vi "mcl_panel_register_events.vi"(8 "error in (no error)":errorcluster, 11 "thorlabs_panel in":refnum<class "mcl_panel.lvclass">) -> (0 "error out":errorcluster, 2 "event_refs cluster":T1, 3 "thorlabs_panel out":refnum<class "mcl_panel.lvclass">)   [LabVIEW 2015, in "mcl_panel.lvclass"]
uses:
  mcl_panel.lvclass
  Thorlabs Kinesis/thorlabs_panel/thorlabs_event_refs.ctl
  Thorlabs Kinesis/thorlabs_panel/thorlabs_events.ctl
  mcl_panel.lvclass/mcl_panel.ctl
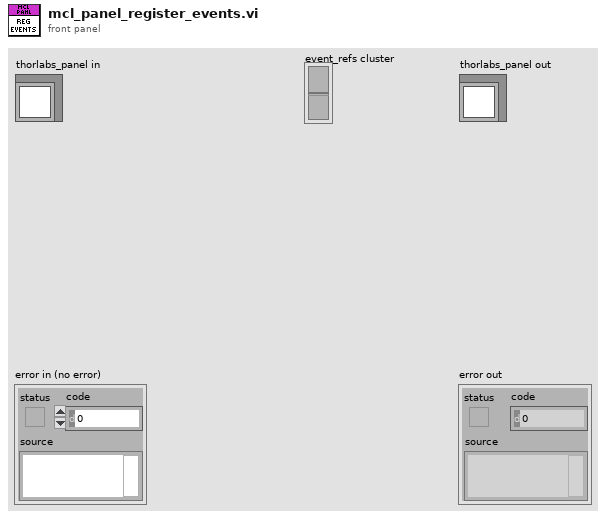
[diagram p1: front panel]
types:
  T1 = typedef "thorlabs_event_refs.ctl" = cluster{"Event Registration Refnum":refnum<event-registration>, "Event Registration Refnum":refnum<event-registration>}
  T2 = typedef "thorlabs_events.ctl" = cluster{"mcl_status":refnum<user-event>, "piezo_positions":refnum<user-event>}
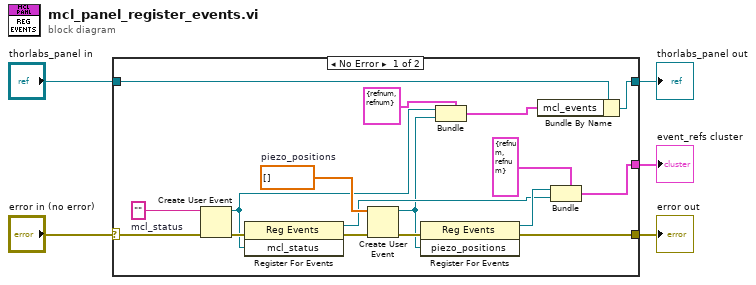
[diagram p0: block diagram]
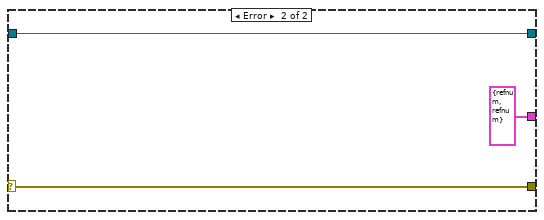
[diagram p2: hidden frame]
diagram:
  n1 = case shown="No Error" "error in (no error)" {
    selector: "error in (no error)" -> [w21 w25]
    tunnel: [w6 w25] -> w4
    tunnel: [w7 w24] -> w2
    tunnel: "thorlabs_panel in" -> [w9 w24]
    tunnel: [w10 T1 {"Event Registration Refnum"=refnum, "Event Registration Refnum"=refnum} ("output cluster")] -> w1
    frame No Error {
      w17 = dbl[] []  # piezo_positions
      w22 = ""  # mcl_status
      n2 = Create User Event(user event datatype=w22, error in=w21) -> (user event=w14:refnum<user-event>, error out=w20:errorcluster)
      n3 = register-events(error in=w20, w14) -> (reference out=w15:refnum<event-registration>, error out=w18:errorcluster)  [unwired: 1 in]
      n4 = Create User Event(user event datatype=w17, error in=w18) -> (user event=w13:refnum<user-event>, error out=w19:errorcluster)
      n5 = register-events(error in=w19, w13) -> (reference out=w16:refnum<event-registration>, error out=w6:errorcluster)  [unwired: 1 in]
      n6 = Bundle(cluster=T2 {"mcl_status"=refnum, "piezo_positions"=refnum} ("output cluster"), "mcl_status"=w14, "piezo_positions"=w13) -> (w8:T2)
      n7 = Bundle By Name(cluster=w9, "mcl_events"=w8) -> (w7:refnum<class "mcl_panel.lvclass">)
      n8 = Bundle(cluster=T1 {"Event Registration Refnum"=refnum, "Event Registration Refnum"=refnum} ("output cluster"), "Event Registration Refnum"=w16, "Event Registration Refnum"=w15) -> (w10:T1)
    }
    frame Error {
    }
  }
  "error out" <- w4
  "thorlabs_panel out" <- w2
  "event_refs cluster" <- w1
